vi "M method (SubVI).vi"(0 "Tc (mSec)":u32 format="%#_6f", 1 "Tick Count (mSec)":u32 format="%#_6f", 2 "Encoder pulses":i32 format="%#_6f", 5 "Shift Register in 1":u32 format="%#_6f", 7 "Shift Register in 2":i32 format="%#_6f", 11 "Encoder velocity_pre (pulse/s)":fxp<+/-,32,25>) -> (6 "Shift Register out 1":u32 format="%#_6f", 8 "Shift Register out 2":i32 format="%#_6f", 15 "Encoder velocity (pulse/s)":fxp<+/-,32,25>)   [LabVIEW 2014]
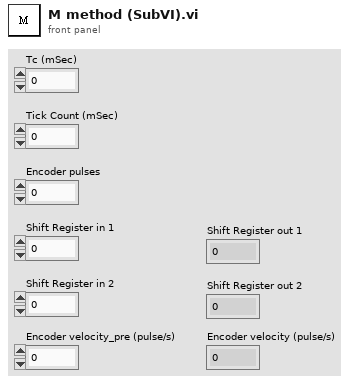
[diagram p1: front panel]
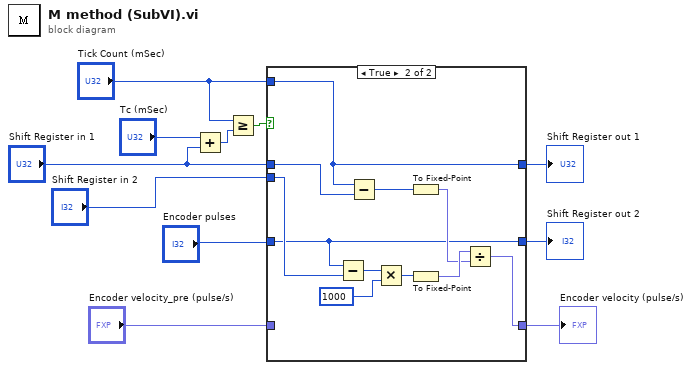
[diagram p0: block diagram]
diagram:
  n1 = Add(x="Tc (mSec)", y="Shift Register in 1") -> (x+y=w4:u32)
  n2 = Greater Or Equal?(x="Tick Count (mSec)", y=w4) -> (x >= y?=w3:bool)
  n3 = case shown="True" w3 {
    tunnel: [w14 w19] -> w5
    tunnel: "Tick Count (mSec)" -> [_ w19]
    tunnel: "Shift Register in 1" -> [w14 w18]
    tunnel: [w13 w15] -> w8
    tunnel: "Encoder pulses" -> [_ w15]
    tunnel: "Shift Register in 2" -> [w13 w17]
    tunnel: "Encoder velocity_pre (pulse/s)" -> [w12 _]
    tunnel: [w12 w16] -> w1
    frame False {
    }
    frame True {
      n4 = Subtract(x=w15, y=w17) -> (x-y=w24:i32)
      n5 = Subtract(x=w19, y=w18) -> (x-y=w25:u32)
      n6 = Multiply(x=w24, y=1000) -> (x*y=w23:i32)
      n7 = To Fixed-Point(number=w25) -> (fixed-point=w21:fxp<+,32,32>)  [unwired: 1 in]
      n8 = To Fixed-Point(number=w23) -> (fixed-point=w22:fxp<+/-,32,32>)  [unwired: 1 in]
      n9 = Divide(x=w22, y=w21) -> (x/y=w16:fxp<+/-,32,25>)
    }
  }
  "Shift Register out 2" <- w8
  "Shift Register out 1" <- w5
  "Encoder velocity (pulse/s)" <- w1
